vi "ATM Messages.vi"(6 "User Input":string, 8 "Error In":errorcluster, 9 "File Data":string[][](array[string]), 10 "Index of Acount":i32, 11 "Atm Message":T1(ring)) -> (0 "error Out":errorcluster, 3 "ATM Messages":string)   [LabVIEW 2024]
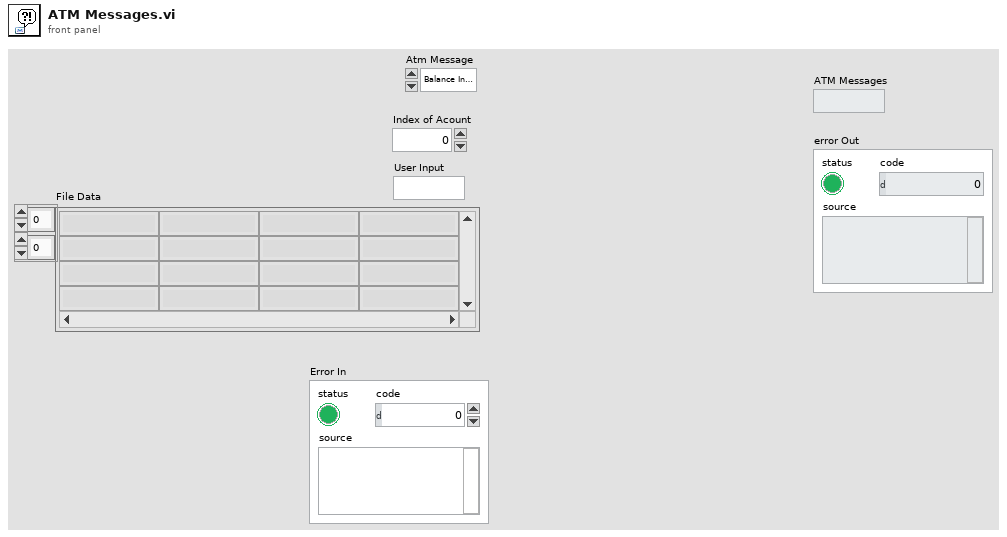
[diagram p1: front panel]
types:
  T1 = enum16{"Balance Inquiry", "Withdrawal Failed", "Withdrawal Complete", "Withdrawal", "Deposit Complete", "Deposit", "Session Terminate", "Account Verification Failed", "Main Menu", "Welcome Message"}
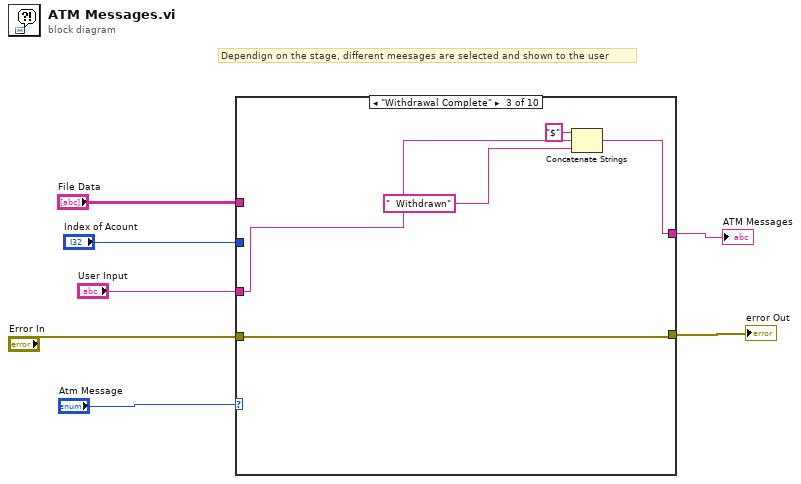
[diagram p0: block diagram]
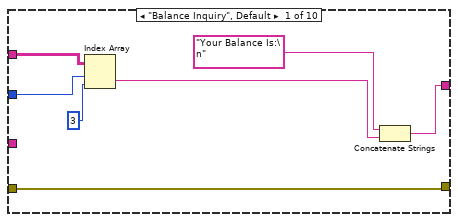
[diagram p2: hidden frame]
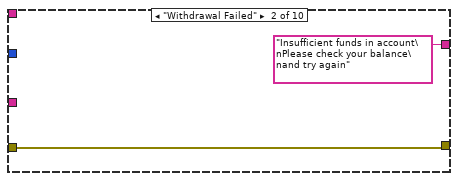
[diagram p3: hidden frame]
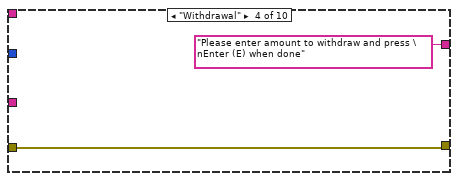
[diagram p4: hidden frame]
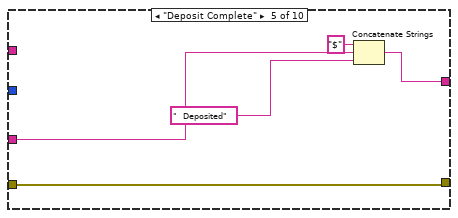
[diagram p5: hidden frame]
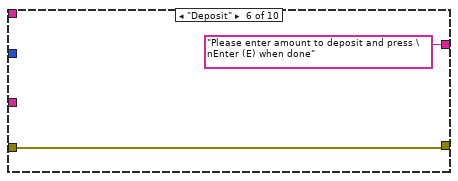
[diagram p6: hidden frame]
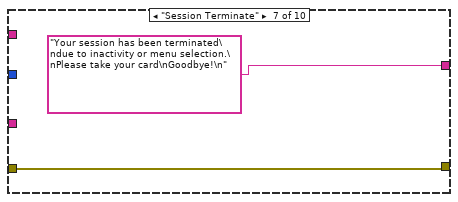
[diagram p7: hidden frame]
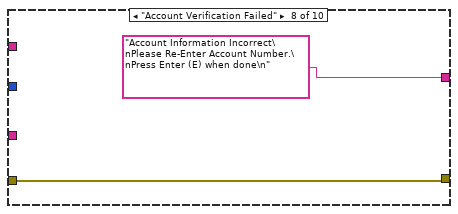
[diagram p8: hidden frame]
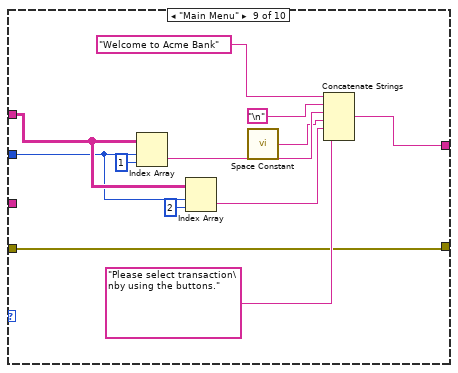
[diagram p9: hidden frame]
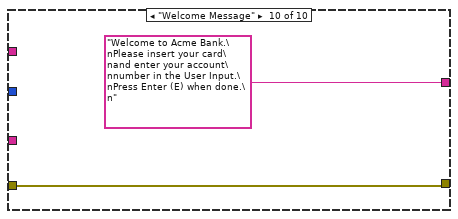
[diagram p10: hidden frame]
diagram:
  # "Dependign on the stage, different meesages are selected and shown to the user"
  n1 = case shown="\"Withdrawal Complete\"" "Atm Message" {
    tunnel: [w8 "Insufficient funds in account\nPlease check your balance\nand try again" ("ATM Messages") w18 "Please enter amount to withdraw and press \nEnter (E) when done" ("ATM Messages") w24 "Please enter amount to deposit and press \nEnter (E) when done" ("ATM Messages") "Your session has been terminated\ndue to inactivity or menu selection.\nPlease take your card\nGoodbye!\n" ("ATM Messages") "Account Information Incorrect\nPlease Re-Enter Account Number.\nPress Enter (E) when done\n" ("ATM Messages") w36 "Welcome to Acme Bank.\nPlease insert your card\nand enter your account\nnumber in the User Input.\nPress Enter (E) when done.\n" ("ATM Messages")] -> w6
    tunnel: "File Data" -> [w12 _ _ _ _ _ _ _ w42 _]
    tunnel: "Index of Acount" -> [w11 _ _ _ _ _ _ _ w41 _]
    tunnel: [w14 w15 w21 w22 w28 w29 w31 w33 w35 w47] -> w3
    tunnel: "Error In" -> [w14 w15 w21 w22 w28 w29 w31 w33 w35 w47]
    tunnel: "User Input" -> [_ _ w17 _ w25 _ _ _ _ _]
    frame "Balance Inquiry", Default {
      n2 = Index Array(array=w12, index (row)=w11, index (col)=3 ("disabled index (col)")) -> (element=w9:string)
      n3 = Concatenate Strings("Your Balance Is:\n" ("ATM Messages"), w9) -> (w8:string)
    }
    frame "Withdrawal Failed" {
    }
    frame "Withdrawal Complete" {
      n4 = Concatenate Strings("$" ("string"), w17, "  Withdrawn" ("ATM Messages")) -> (w18:string)
    }
    frame "Withdrawal" {
    }
    frame "Deposit Complete" {
      n5 = Concatenate Strings("$" ("string"), w25, "  Deposited" ("ATM Messages")) -> (w24:string)
    }
    frame "Deposit" {
    }
    frame "Session Terminate" {
    }
    frame "Account Verification Failed" {
    }
    frame "Main Menu" {
      n6 = Index Array(array=w42, index (row)=w41, index (col)=1 ("disabled index (col)")) -> (element=w44:string)
      n7 = Index Array(array=w42, index (row)=w41, index (col)=2 ("disabled index (col)")) -> (element=w38:string)
      n8 = call <vilib>:"Space Constant.vi"() -> ("String"=w39:string)
      n9 = Concatenate Strings("Welcome to Acme Bank" ("string"), "\n", w44, w39, w38, "Please select transaction\nby using the buttons." ("ATM Messages")) -> (w36:string)
    }
    frame "Welcome Message" {
    }
  }
  "ATM Messages" <- w6
  "error Out" <- w3
